vi "initilize.vi"(8 "error in (no error)":errorcluster, 9 "Serial device Brand":T1, 10 "VISA resource name":refnum<visa-resource-name>, 11 "Serial Device in":refnum<class "Serial Device.lvclass">) -> (0 "error out":errorcluster, 3 "Serial Device out":refnum<class "Serial Device.lvclass">)   [LabVIEW 2019, in "Serial Device.lvclass"]
uses:
  Serial Device.lvclass
  Control 14.ctl
  <vilib>/Instr/_visa.llb/VISA Configure Serial Port (Instr).vi
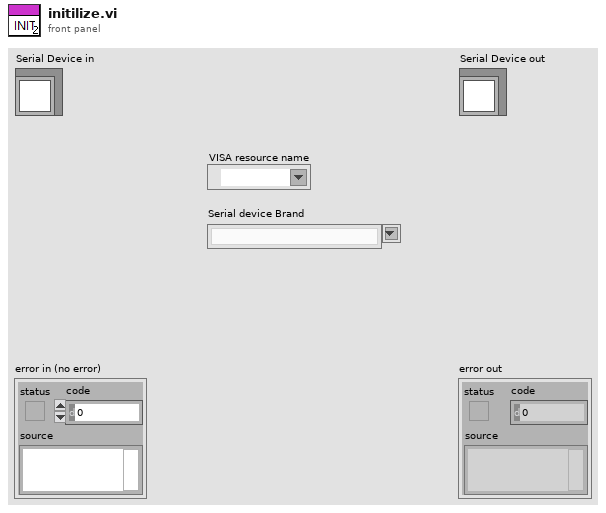
[diagram p1: front panel]
types:
  T1 = typedef "Serial Device.lvclass/Control 14.ctl" = string
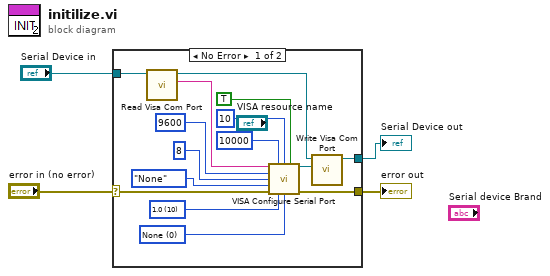
[diagram p0: block diagram]
diagram:
  n1 = case shown="No Error" "error in (no error)" {
    selector: "error in (no error)" -> [w14 w21]
    tunnel: [w13 w21] -> w3
    tunnel: [w15 w20] -> w1
    tunnel: "Serial Device in" -> [w17 w20]
    frame No Error {
      w5 = u16 0 items=["None", "XON/XOFF", "RTS/CTS", "XON/XOFF & RTS/CTS", "DTR/DSR", "XON/XOFF & DTR/DSR"] ("flow control (0:none)")
      w6 = u16 10 items=["1.0"=10, "1.5"=15, "2.0"=20] ("stop bits (10: 1 bit)")
      n2 = call-dynamic "Read Visa Com Port.vi"("Serial Device in"=w17) -> ("Visa Com Port"=w19:string, "Serial Device out"=w16:refnum<class "Serial Device.lvclass">)  [unwired: 8 in, 1 out]
      n3 = call-poly "VISA Configure Serial Port"("VISA resource name"=w19, "timeout (10sec)"=u32 10000, "termination char\n(0xA = '\\n' = LF)"=u8 10 ("termination char\n(0xA = '\\n' = LF)"), "Enable Termination\nChar (T)"=TRUE ("Enable Termination\nChar (T)"), "baud rate (9600)"=u32 9600, "data bits (8)"=u16 8, "parity (0:none)"=enum16{"None", "Odd", "Even", "Mark", "Space"}."None", "error in (no error)"=w14, "stop bits (10: 1 bit)"=w6, "flow control (0:none)"=w5) -> ("VISA resource name out"=w18:refnum<visa-resource-name>, "error out"=w13:errorcluster)  [unwired: 4 in]
      n4 = call-dynamic "Write Visa Com Port.vi"("Visa Com Port"=w18, "Serial Device in"=w16) -> ("Serial Device out"=w15:refnum<class "Serial Device.lvclass">)  [unwired: 8 in, 1 out]
    }
    frame Error {
    }
  }
  "error out" <- w3
  "Serial Device out" <- w1
